vi "Get Label.vi"(8 "error in (no error)":errorcluster, 11 "Search in":refnum<class "Search.lvclass">) -> (0 "error out":errorcluster, 2 "Label":string, 3 "Search out":refnum<class "Search.lvclass">)   [LabVIEW 2016, in "Better Search.lvlib" / "Search.lvclass"]
uses:
  Search.lvclass
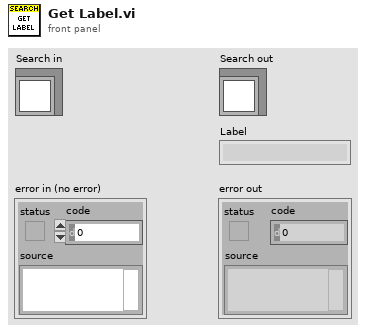
[diagram p1: front panel]
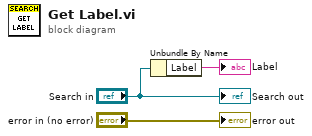
[diagram p0: block diagram]
diagram:
  n1 = Unbundle By Name("Search in") -> ("Label"=→"Label":string)
  "error out" <- "error in (no error)"
  "Search out" <- "Search in"
